vi "TestUI.vi"(0 "Control9":csg, 1 "Text1":string, 5 "Control1":dbl, 9 "Boolean":bool, 11 "Array":dbl[](array[numeric])) -> ()   [LabVIEW 2016]
panel:
  in  "Table Control":string[][](table)
  in  "Numeric 2":dbl
  in  "Numeric":i32
  in  "Path":path
  in  "Tab Control":enum32{"Page 1", "Page 2", "Page 3"}(tab)
  in  "Slide":dbl(slide) scale=0.0..10.0
  in  "Control5":i32
  in  "Control4":csg
  in  "String1":string
  out "Meter":dbl(knob) scale=0.0..10.0
  out "Slide 2":u8(slide) scale=0.0..100.0
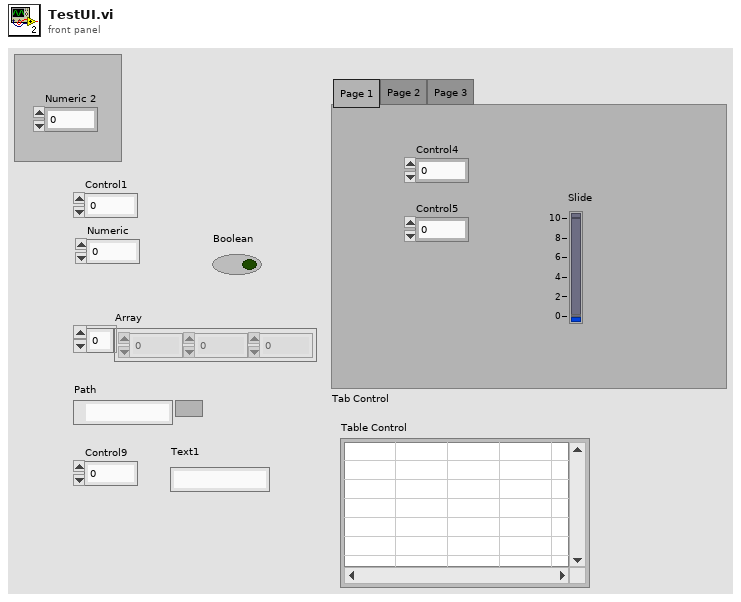
[diagram p1: front panel]
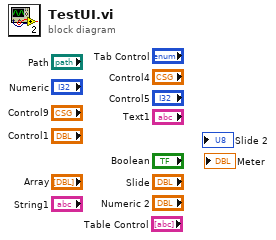
[diagram p0: block diagram]
diagram:
